vi "Teleop - Shooter Manual Control (SubVI).vi"(7 "Desired cluster In":T1 {"shooterMotorMode" items=["PercentOutput"=0, "Position"=1, "Velocity"=2, "Current"=3, "Follower"=5, "MotionProfile"=6, "MotionMagic"=7, "MotionProfileArc"=10, "Disabled"=15]}, 9 "Constant Cluster in":T3 {"12. Auton Deriv Drive Straight Gain" format="%_6f"; "11. Auton Int Drive Straight Gain" format="%_6f"; "10. Auton Prop Drive Straight Gain" format="%_6f"; "9. Auton I Output Limit Turn Gain" format="%_6f"; "8. Auton Deriv Turn Gain" format="%_6f"; "7. Auton Int Turn Gain" format="%_6f"; "1. Auton Prop Drive Gain" format="%_6f"; "2. Auton Int Drive Gain" format="%_6f"; "3. Auton Deriv Drive Gain" format="%_6f"; "4. I Output Drive  Limit" format="%_6f"; "5. Auto Drive Cheat (%)" format="%_6f"; "6. Auton Prop Turn Gain" format="%_6f"}, 11 "sensors In":T4, 12 "manual-buttonPress?":bool) -> (8 "Desired cluster Out":T1 {"shooterMotorMode" items=["PercentOutput"=0, "Position"=1, "Velocity"=2, "Current"=3, "Follower"=5, "MotionProfile"=6, "MotionMagic"=7, "MotionProfileArc"=10, "Disabled"=15]}, 10 "Constant Cluster Out":T3 {"12. Auton Deriv Drive Straight Gain" format="%_6f"; "11. Auton Int Drive Straight Gain" format="%_6f"; "10. Auton Prop Drive Straight Gain" format="%_6f"; "9. Auton I Output Limit Turn Gain" format="%_6f"; "8. Auton Deriv Turn Gain" format="%_6f"; "7. Auton Int Turn Gain" format="%_6f"; "1. Auton Prop Drive Gain" format="%_6f"; "2. Auton Int Drive Gain" format="%_6f"; "3. Auton Deriv Drive Gain" format="%_6f"; "4. I Output Drive  Limit" format="%_6f"; "5. Auto Drive Cheat (%)" format="%_6f"; "6. Auton Prop Turn Gain" format="%_6f"}, 15 "sensors Out":T4)   [LabVIEW 2019]
uses:
  Autonomous/TypeDefs/Sensor TypeDef.ctl
  Disabled/Constant VI_s/Disabled - Constant Cluster Typedef.ctl
  Desired Cluster.ctl
  <vilib>/Rock Robotics/WPI/ThirdParty/Phoenix-LabVIEW/Motor Controller/Controls/CTRE_Phoenix_MotorControl_ControlMode.ctl
panel:
  in  "Manual Hood Gain":dbl
  in  "Manual Turret Gain":dbl
  in  "Right Joy Y Axis":dbl
  in  "Left Joy X Axis":dbl
  # "Inputs"
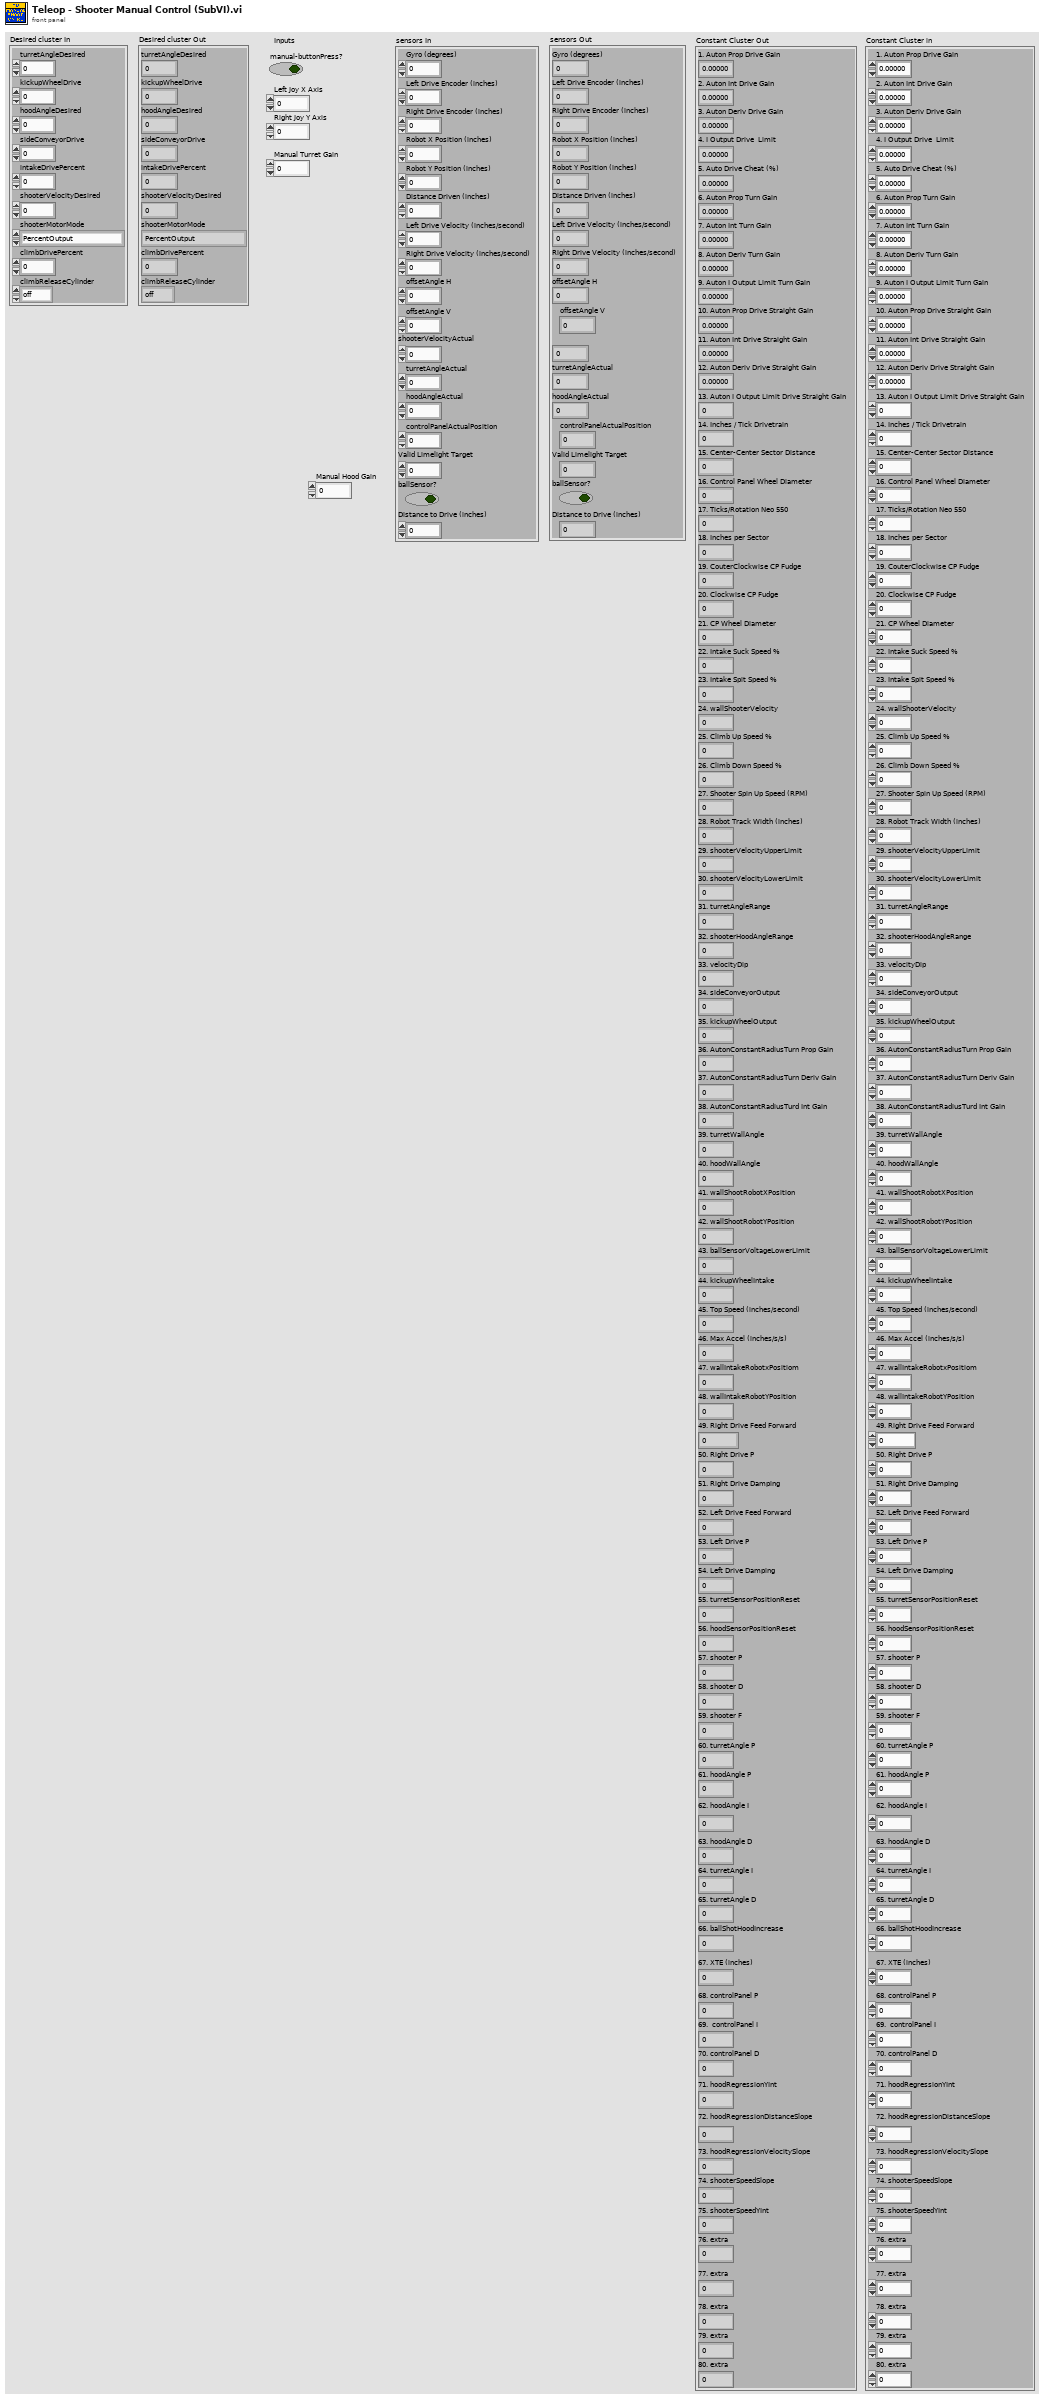
[diagram p1: front panel]
types:
  T1 = typedef "Desired Cluster.ctl" = cluster{"turretAngleDesired":dbl, "kickupWheelDrive":dbl, "hoodAngleDesired":dbl, "sideConveyorDrive":dbl, "intakeDrivePercent":dbl, "shooterVelocityDesired":dbl, "shooterMotorMode":T2, "climbDrivePercent":dbl, "climbReleaseCylinder":enum16{"off", "on", "forward", "back"}}
  T2 = typedef "CTRE_Phoenix_MotorControl_ControlMode.ctl" = u16
  T3 = typedef "Disabled - Constant Cluster Typedef.ctl" = cluster{"1. Auton Prop Drive Gain":dbl, "2. Auton Int Drive Gain":dbl, "3. Auton Deriv Drive Gain":dbl, "4. I Output Drive  Limit":dbl, "5. Auto Drive Cheat (%)":dbl, "6. Auton Prop Turn Gain":dbl, "7. Auton Int Turn Gain":dbl, "8. Auton Deriv Turn Gain":dbl, "9. Auton I Output Limit Turn Gain":dbl, "10. Auton Prop Drive Straight Gain":dbl, "11. Auton Int Drive Straight Gain":dbl, "12. Auton Deriv Drive Straight Gain":dbl, "13. Auton I Output Limit Drive Straight Gain":dbl, "14. Inches / Tick Drivetrain":dbl, "15. Center-Center Sector Distance":dbl, "16. Control Panel Wheel Diameter":dbl, "17. Ticks/Rotation Neo 550":dbl, "18. Inches per Sector":dbl, "19. CouterClockwise CP Fudge":dbl, "20. Clockwise CP Fudge":dbl, "21. CP Wheel Diameter":dbl, "22. Intake Suck Speed %":dbl, "23. Intake Spit Speed %":dbl, "24. wallShooterVelocity":dbl, "25. Climb Up Speed %":dbl, "26. Climb Down Speed %":dbl, "27. Shooter Spin Up Speed (RPM)":dbl, "28. Robot Track Width (inches)":dbl, "29. shooterVelocityUpperLimit":dbl, "30. shooterVelocityLowerLimit":dbl, "31. turretAngleRange":dbl, "32. shooterHoodAngleRange":dbl, "33. velocityDip":dbl, "34. sideConveyorOutput":dbl, "35. kickupWheelOutput":dbl, "36. AutonConstantRadiusTurn Prop Gain":dbl, "37. AutonConstantRadiusTurn Deriv Gain":dbl, "38. AutonConstantRadiusTurd Int Gain":dbl, "39. turretWallAngle":dbl, "40. hoodWallAngle":dbl, "41. wallShootRobotXPosition":dbl, "42. wallShootRobotYPosition":dbl, "43. ballSensorVoltageLowerLimit":dbl, "44. kickupWheelIntake":dbl, "45. Top Speed (inches/second)":dbl, "46. Max Accel (inches/s/s)":dbl, "47. wallIntakeRobotxPositiom":dbl, "48. wallIntakeRobotYPosition":dbl, "49. Right Drive Feed Forward":dbl, "50. Right Drive P":dbl, "51. Right Drive Damping":dbl, "52. Left Drive Feed Forward":dbl, "53. Left Drive P":dbl, "54. Left Drive Damping":dbl, "55. turretSensorPositionReset":dbl, "56. hoodSensorPositionReset":dbl, "57. shooter P":dbl, "58. shooter D":dbl, "59. shooter F":dbl, "60. turretAngle P":dbl, "61. hoodAngle P":dbl, "62. hoodAngle I":dbl, "63. hoodAngle D":dbl, "64. turretAngle I":dbl, "65. turretAngle D":dbl, "66. ballShotHoodIncrease":dbl, "67. XTE (inches)":dbl, "68. controlPanel P":dbl, "69.  controlPanel I":dbl, "70. controlPanel D":dbl, "71. hoodRegressionYInt":dbl, "72. hoodRegressionDistanceSlope":dbl, "73. hoodRegressionVelocitySlope":dbl, "74. shooterSpeedSlope":dbl, "75. shooterSpeedYInt":dbl, "76. extra":dbl, "77. extra":dbl, "78. extra":dbl, "79. extra":dbl, "80. extra":dbl}
  T4 = typedef "Sensor TypeDef.ctl" = cluster{"Gyro (degrees)":dbl, "Left Drive Encoder (inches)":dbl, "Right Drive Encoder (inches)":dbl, "Robot X Position (inches)":dbl, "Robot Y Position (inches)":dbl, "Distance Driven (inches)":dbl, "Left Drive Velocity (inches/second)":dbl, "Right Drive Velocity (inches/second)":dbl, "offsetAngle H":dbl, "offsetAngle V":dbl, "shooterVelocityActual":dbl, "turretAngleActual":dbl, "hoodAngleActual":dbl, "controlPanelActualPosition":dbl, "Valid Limelight Target":dbl, "ballSensor?":bool, "Distance to Drive (inches)":dbl}
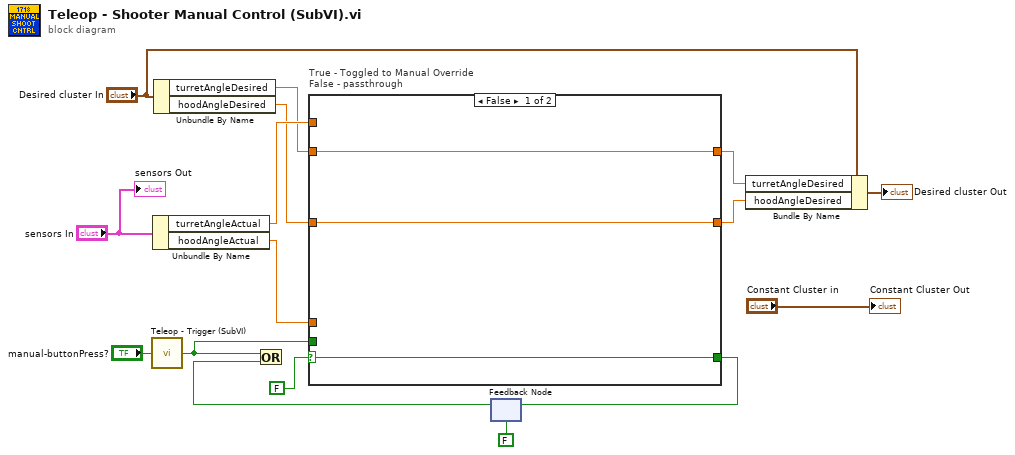
[diagram p0: block diagram]
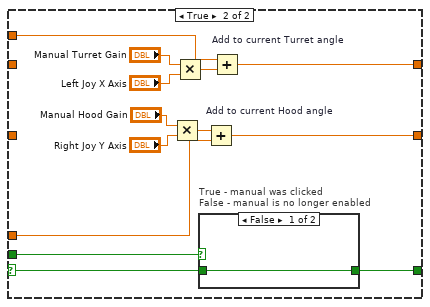
[diagram p2: hidden frame]
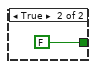
[diagram p3: hidden frame]
diagram:
  n1 = call "Teleop - Trigger (SubVI).vi"("Trigger"="manual-buttonPress?") -> ("Trigger Output"=w12:bool)
  n2 = Unbundle By Name("sensors In") -> ("turretAngleActual"=w10:dbl, "hoodAngleActual"=w9:dbl)
  n3 = Unbundle By Name("Desired cluster In") -> ("turretAngleDesired"=w6:dbl, "hoodAngleDesired"=w5:dbl)
  n4 = case "True - Toggled to Manual Override\nFalse - passthrough" shown="False" FALSE {
    selector: FALSE -> [w17 w20]
    tunnel: w10 -> [_ w26]
    tunnel: w9 -> [_ w25]
    tunnel: [w18 w24] -> w1
    tunnel: [w19 w23] -> w2
    tunnel: w6 -> [w19 _]
    tunnel: w5 -> [w18 _]
    tunnel: [w17 w21] -> w16
    tunnel: w12 -> [_ w22]
    frame False {
    }
    frame True {
      n5 = Multiply(x="Manual Hood Gain", y="Right Joy Y Axis") -> (x*y=w31:dbl)
      n6 = Multiply(x="Manual Turret Gain", y="Left Joy X Axis") -> (x*y=w29:dbl)
      n7 = case "True - manual was clicked\nFalse - manual is no longer enabled" shown="False" w22 {
        tunnel: [w33 FALSE] -> w21
        tunnel: w20 -> [w33 _]
        frame False {
        }
        frame True {
        }
      }
      n8 = Add "Add to current Hood angle"(x=w31, y=w25) -> (x+y=w24:dbl)
      n9 = Add "Add to current Turret angle"(x=w26, y=w29) -> (x+y=w23:dbl)
    }
  }
  n10 = feedback-in #1(w16) -> ()
  n11 = feedback #1(FALSE) -> (w14:bool)
  n12 = Or(x=w12, y=w14) -> ()  [unwired: 1 out]
  n13 = Bundle By Name(cluster="Desired cluster In", "turretAngleDesired"=w2, "hoodAngleDesired"=w1) -> (→"Desired cluster Out":T1)
  "sensors Out" <- "sensors In"
  "Constant Cluster Out" <- "Constant Cluster in"
